vi "InternalStacking.vi"() -> ()   [LabVIEW 2014]
uses:
  InternalStacking.ctl
  <vilib>/Rock Robotics/WPI/Joystick/WPI_JoystickGetSetRefNum.vi
panel:
  in  "State of Elevator":T1
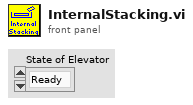
[diagram p1: front panel]
types:
  T1 = typedef "InternalStacking.ctl" = enum16{"Ready", "Extend Plate", "Lift Tote", "Wait For Seated Tote", "Release Tote", "Reset To Bottom Limit "}
  T2 = typedef "WPI_JoystickDevRef.ctl" = cluster{"Device":T3}
  T3 = typedef "WPI_JoystickDeviceEnum.ctl" = enum16{"USB 0", "USB 1", "USB 2", "USB 3", "USB 4", "USB 5"}
  T4 = cluster{"Buttons[0]":bool, "Buttons[1]":bool, "Buttons[2]":bool, "Buttons[3]":bool, "Buttons[4]":bool, "Buttons[5]":bool, "Buttons[6]":bool, "Buttons[7]":bool, "Buttons[8]":bool}
  T5 = typedef "WPI_ServoDeviceRef.ctl" = cluster{"DeviceStatus":errorcluster, "Controller":T6, "PWM Channel":T7, "DeadBand":T8}
  T6 = typedef "FPGA_TypedefDigitalModule.ctl" = enum16{"Controller 1"}
  T7 = typedef "FPGA_DIOPWMChannel.ctl" = enum8{"PWM 0", "PWM 1", "PWM 2", "PWM 3", "PWM 4", "PWM 5", "PWM 6", "PWM 7", "PWM 8", "PWM 9", "PWM MXP 0", "PWM MXP 1", "PWM MXP 2", "PWM MXP 3", "PWM MXP 4", "PWM MXP 5", "PWM MXP 6", "PWM MXP 7", "PWM MXP 8", "PWM MXP 9", "Invalid"}
  T8 = typedef "WPI_PWMDeadband.ctl" = cluster{"Name":string, "maxPositivePwm":i32, "minPositivePwm":i32, "centerPwm":i32, "maxNegativePwm":i32, "minNegativePwm":i32, "angularRange":u16}
  T9 = typedef "WPI_DigitalInputDevRef.ctl" = cluster{"DevStatus":errorcluster, "DIO Channel":T10, "Controller":T6}
  T10 = typedef "FPGA_DIOChannel.ctl" = enum8{"DIO 0", "DIO 1", "DIO 2", "DIO 3", "DIO 4", "DIO 5", "DIO 6", "DIO 7", "DIO 8", "DIO 9", "DIO MXP 0", "DIO MXP 1", "DIO MXP 2", "DIO MXP 3", "DIO MXP 4", "DIO MXP 5", "DIO MXP 6", "DIO MXP 7", "DIO MXP 8", "DIO MXP 9", "DIO MXP 10", "DIO MXP 11", "DIO MXP 12", "DIO MXP 13", "DIO MXP 14", "DIO MXP 15", "Invalid"}
  T11 = typedef "WPI_MotorControlDeviceRef.ctl" = cluster{"DeviceStatus":errorcluster, "Type":T12, "PWM":cluster{"Controller":T6, "PWM Channel":T7, "DeadBand":T8}, "CAN":cluster{"Device Number":u8, "Control Mode":T13, "Semaphore":T14, "Max Vout":dbl, "TalonSRX Control Mode":T15}, "Invert":bool, "TransformRef":T16, "InvTransformRef":T16}
  T12 = typedef "WPI_MotorControlType.ctl" = enum16{"PWM", "CAN", "CANTalonSRX"}
  T13 = typedef "WPI_CANJaguar_ControlMode.ctl" = enum8{"Percent VBus", "Current", "Speed", "Position", "Voltage"}
  T14 = typedef "Semaphore RefNum" = refnum<k1>
  T15 = typedef "WPI_CANTalonSRX_APIControlMode.ctl" = enum8{"Percent VBus", "Speed", "Position", "Slave", "Unchanged / Invalid"}
  T16 = typedef "WPI_PWMTransform_ConPane.ctl" = refnum<vi>
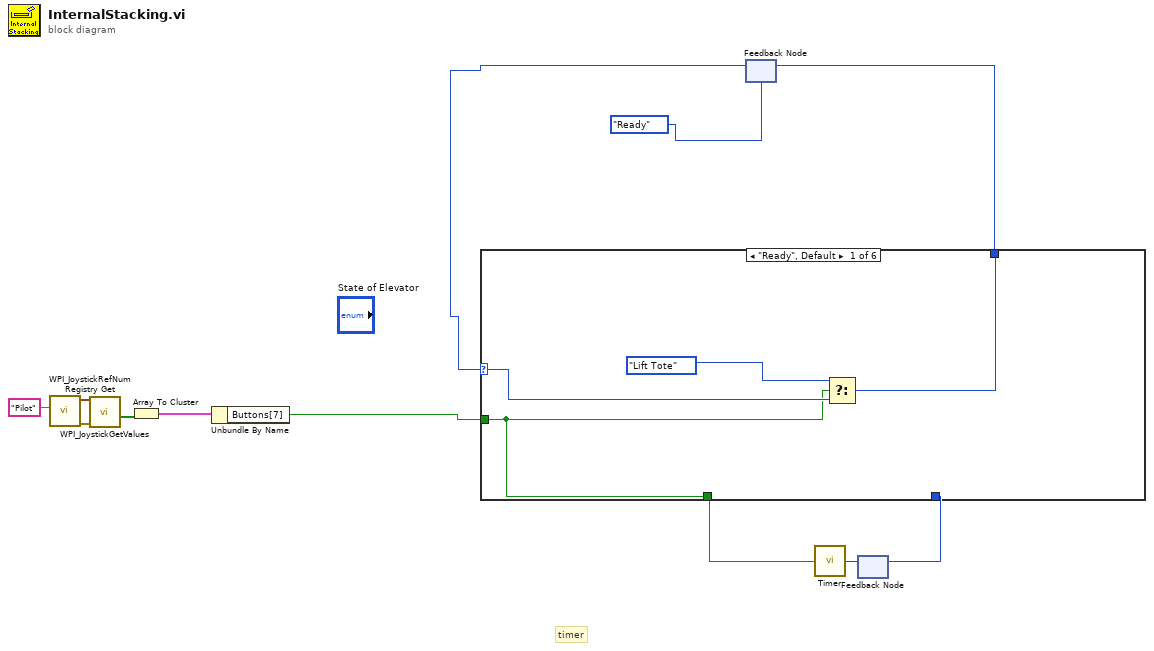
[diagram p0: block diagram]
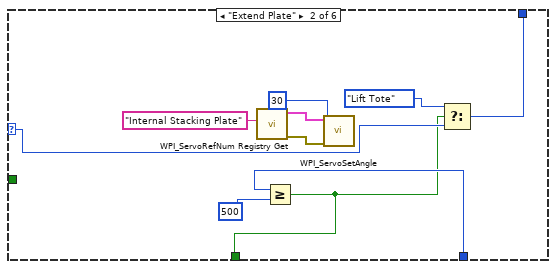
[diagram p2: hidden frame]
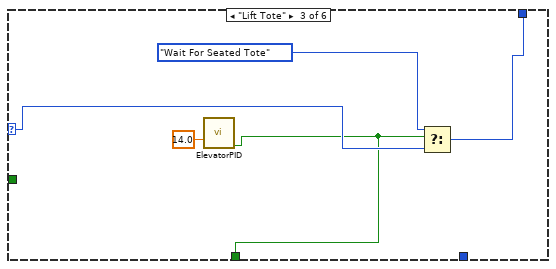
[diagram p3: hidden frame]
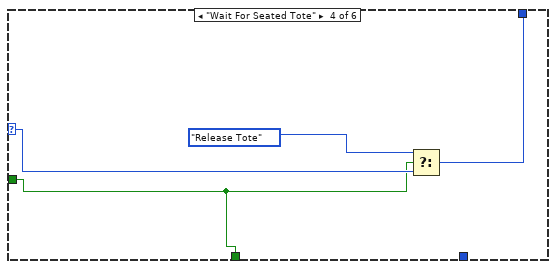
[diagram p4: hidden frame]
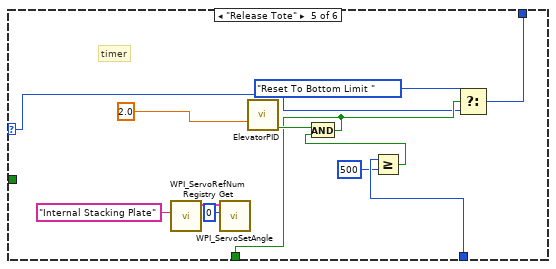
[diagram p5: hidden frame]
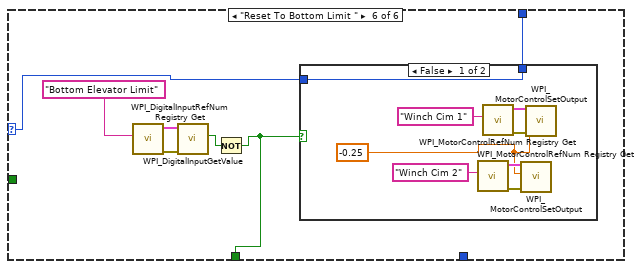
[diagram p6: hidden frame]
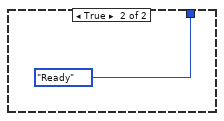
[diagram p7: hidden frame]
diagram:
  # "timer"
  n1 = call <vilib>:"WPI_JoystickRefNum Registry Get.vi"("refnum name"="Pilot") -> ("error out"=w11:errorcluster, "JoystickDevRef"=w10:T2)  [unwired: 9 in]
  n2 = call <vilib>:"WPI_JoystickGetValues.vi"("error in (no error)"=w11, "JoystickDevRef"=w10) -> ("Buttons"=w9:bool[])  [unwired: 5 in, 4 out]
  n3 = Array To Cluster(array=w9) -> (cluster=w8:T4)
  n4 = Unbundle By Name(w8) -> ("Buttons[7]"=w5:bool)
  n5 = feedback #1(InternalStacking."Ready" ("State of Elevator")) -> (w6:T1)
  n6 = feedback #2() -> (w1:u64)  [unwired: 1 in]
  n7 = case shown="\"Ready\", Default" w6 {
    selector: w6 -> [w15 w21 w29 w34 w38 w49]
    tunnel: w5 -> [w13 _ _ w32 _ _]
    tunnel: [w14 w20 w28 w33 w36 w50] -> w4
    tunnel: [w13 w17 w27 w32 w39 w48] -> w3
    tunnel: w1 -> [_ w19 _ _ w42 _]
    frame "Ready", Default {
      n8 = Select(t=InternalStacking."Lift Tote" ("State of Elevator"), s=w13, f=w15) -> (s? t:f=w14:T1)
    }
    frame "Extend Plate" {
      n9 = call <vilib>:"WPI_ServoRefNum Registry Get.vi"("refnum name"="Internal Stacking Plate") -> ("error out"=w25:errorcluster, "ServoDeviceRef"=w24:T5)  [unwired: 9 in]
      n10 = Greater Or Equal?(x=w19, y=500) -> (x >= y?=w17:bool)
      n11 = call <vilib>:"WPI_ServoSetAngle.vi"("error in (no error)"=w25, "Angle"=30, "ServoDeviceRef"=w24) -> ()  [unwired: 7 in, 2 out]
      n12 = Select(t=InternalStacking."Lift Tote" ("State of Elevator"), s=w17, f=w21) -> (s? t:f=w20:T1)
    }
    frame "Lift Tote" {
      n13 = call "ElevatorPID.vi"("Elevator Setpoint"=14.0) -> ("At Setpoint"=w27:bool)  [unwired: 14 in]
      n14 = Select(t=InternalStacking."Wait For Seated Tote" ("State of Elevator"), s=w27, f=w29) -> (s? t:f=w28:T1)
    }
    frame "Wait For Seated Tote" {
      n15 = Select(t=InternalStacking."Release Tote" ("State of Elevator"), s=w32, f=w34) -> (s? t:f=w33:T1)
    }
    frame "Release Tote" {
      # "timer"
      n16 = call <vilib>:"WPI_ServoRefNum Registry Get.vi"("refnum name"="Internal Stacking Plate") -> ("ServoDeviceRef"=w44:T5)  [unwired: 9 in, 1 out]
      n17 = call <vilib>:"WPI_ServoSetAngle.vi"("Angle"=0, "ServoDeviceRef"=w44) -> ()  [unwired: 8 in, 2 out]
      n18 = call "ElevatorPID.vi"("Elevator Setpoint"=2.0) -> ("At Setpoint"=w46:bool)  [unwired: 14 in]
      n19 = Greater Or Equal?(x=w42, y=u64 500) -> (x >= y?=w40:bool)
      n20 = And(x=w46, y=w40) -> (x .and. y?=w39:bool)
      n21 = Select(t=InternalStacking."Reset To Bottom Limit " ("State of Elevator"), s=w39, f=w38) -> (s? t:f=w36:T1)
    }
    frame "Reset To Bottom Limit " {
      n22 = call <vilib>:"WPI_DigitalInputRefNum Registry Get.vi"("refnum name"="Bottom Elevator Limit") -> ("error out"=w53:errorcluster, "DigitalInputDevRef"=w52:T9)  [unwired: 9 in]
      n23 = call <vilib>:"WPI_DigitalInputGetValue.vi"("error in (no error)"=w53, "DigitalInputDevRef"=w52) -> ("Value"=w51:bool)  [unwired: 7 in, 2 out]
      n24 = Not(x=w51) -> (.not. x?=w48:bool)
      n25 = case shown="False" w48 {
        tunnel: [w56 InternalStacking."Ready" ("State of Elevator")] -> w50
        tunnel: w49 -> [w56 _]
        frame False {
          w55 = -0.25 ("Output")
          n26 = call <vilib>:"WPI_MotorControlRefNum Registry Get.vi"("refnum name"="Winch Cim 2") -> ("error out"=w58:errorcluster, "MotorControlDevRef"=w57:T11)  [unwired: 9 in]
          n27 = call <vilib>:"WPI_MotorControlRefNum Registry Get.vi"("refnum name"="Winch Cim 1") -> ("error out"=w61:errorcluster, "MotorControlDevRef"=w60:T11)  [unwired: 9 in]
          n28 = call <vilib>:"WPI_MotorControlSetOutput.vi"("error in (no error)"=w58, "Output"=w55, "MotorControlDevRef"=w57) -> ()  [unwired: 6 in, 3 out]
          n29 = call <vilib>:"WPI_MotorControlSetOutput.vi"("error in (no error)"=w61, "Output"=w55, "MotorControlDevRef"=w60) -> ()  [unwired: 6 in, 3 out]
        }
        frame True {
        }
      }
    }
  }
  n30 = feedback-in #1(w4) -> ()
  n31 = call "Timer.vi"("Set Timer"=w3) -> ("Time elapsed"=w2:u64)
  n32 = feedback-in #2(w2) -> ()
